vi "notifier ex- 2.vi"() -> ()   [LabVIEW 2022 SP3]
panel:
  in  "stop 3":bool
  in  "stop 2":bool
  in  "stop":bool
  out "Waveform Chart 3":dbl(graph)
  out "Waveform Chart 2":dbl(graph)
  out "Waveform Chart":dbl(graph)
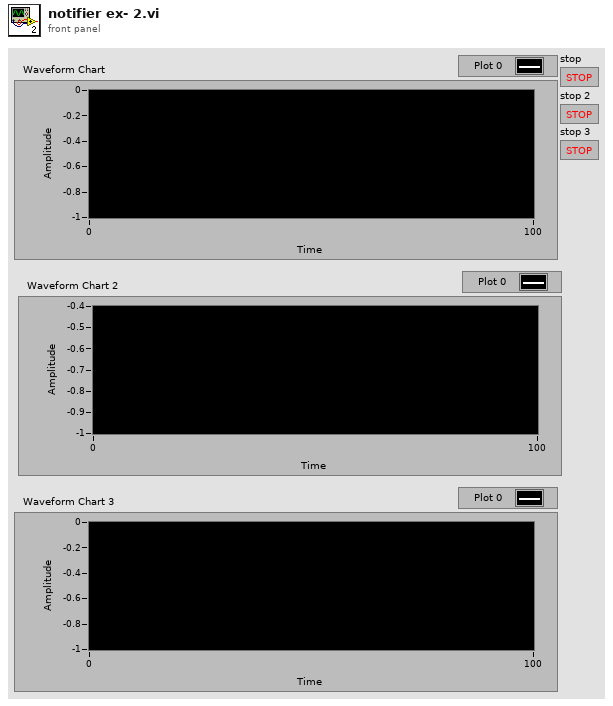
[diagram p1: front panel]
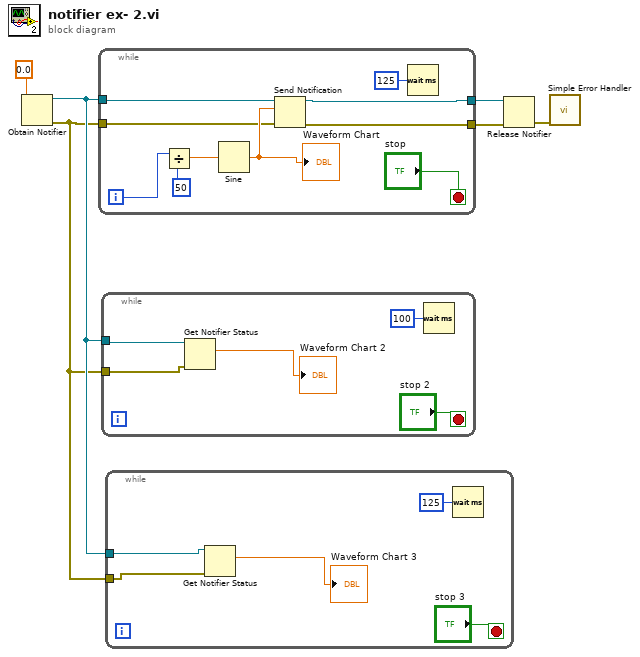
[diagram p0: block diagram]
diagram:
  n1 = Obtain Notifier(notification data type=0.0) -> (notifier out=w5:refnum<notifier>, error out=w4:errorcluster)  [unwired: 3 in, 1 out]
  n2 = while {
    tunnel: w5 -> [w10]
    tunnel: w4 -> [w9]
    tunnel: [w8] -> w2
    tunnel: [w7] -> w3
    i -> [w16]
    stop <- "stop" stop-if-true
    n3 = Divide(x=w16, y=50) -> (x/y=w14:dbl)
    n4 = Sine(x=w14) -> (sin(x)=w11:dbl)
    "Waveform Chart" <- w11
    n5 = Send Notification(notification=w11, notifier=w10, error in (no error)=w9) -> (notifier out=w8:refnum<notifier>, error out=w7:errorcluster)
    n6 = Wait (ms)(milliseconds to wait=u32 125) -> ()  [unwired: 1 out]
  }
  n7 = while {
    tunnel: w5 -> [w20]
    tunnel: w4 -> [w19]
    stop <- "stop 2" stop-if-true
    n8 = Get Notifier Status(notifier=w20, error in (no error)=w19) -> (current notification=→"Waveform Chart 2":dbl)  [unwired: 4 out]
    n9 = Wait (ms)(milliseconds to wait=u32 100) -> ()  [unwired: 1 out]
  }
  n10 = while {
    tunnel: w5 -> [w25]
    tunnel: w4 -> [w24]
    stop <- "stop 3" stop-if-true
    n11 = Get Notifier Status(notifier=w25, error in (no error)=w24) -> (current notification=→"Waveform Chart 3":dbl)  [unwired: 4 out]
    n12 = Wait (ms)(milliseconds to wait=u32 125) -> ()  [unwired: 1 out]
  }
  n13 = Release Notifier(notifier=w2, error in (no error)=w3) -> (error out=w1:errorcluster)  [unwired: 1 in, 2 out]
  n14 = call <vilib>:"Simple Error Handler.vi"("error in (no error)"=w1) -> ()  [unwired: 4 in, 5 out]
